vi "welcome.vi"() -> ()   [LabVIEW 2017]
uses:
  GLOBAL/auto.vi
  GLOBAL/all vi close.vi
panel:
  out "first time direct auto":bool
  in  "error in":errorcluster
  in  "EXIT":bool
  in  "PRINTER":bool
  in  "DATA\nHISTORY":bool
  in  "MAIN":bool
  in  "LOGOUT":bool
  in  "USER":bool
  in  "COUNTER":bool
  in  "SETTING":bool
  in  "SHIFT SETTING":bool
  in  "LOGIN":bool
  # "TRACEABILITY"
  # "Powered By- NI Vision, Pune"
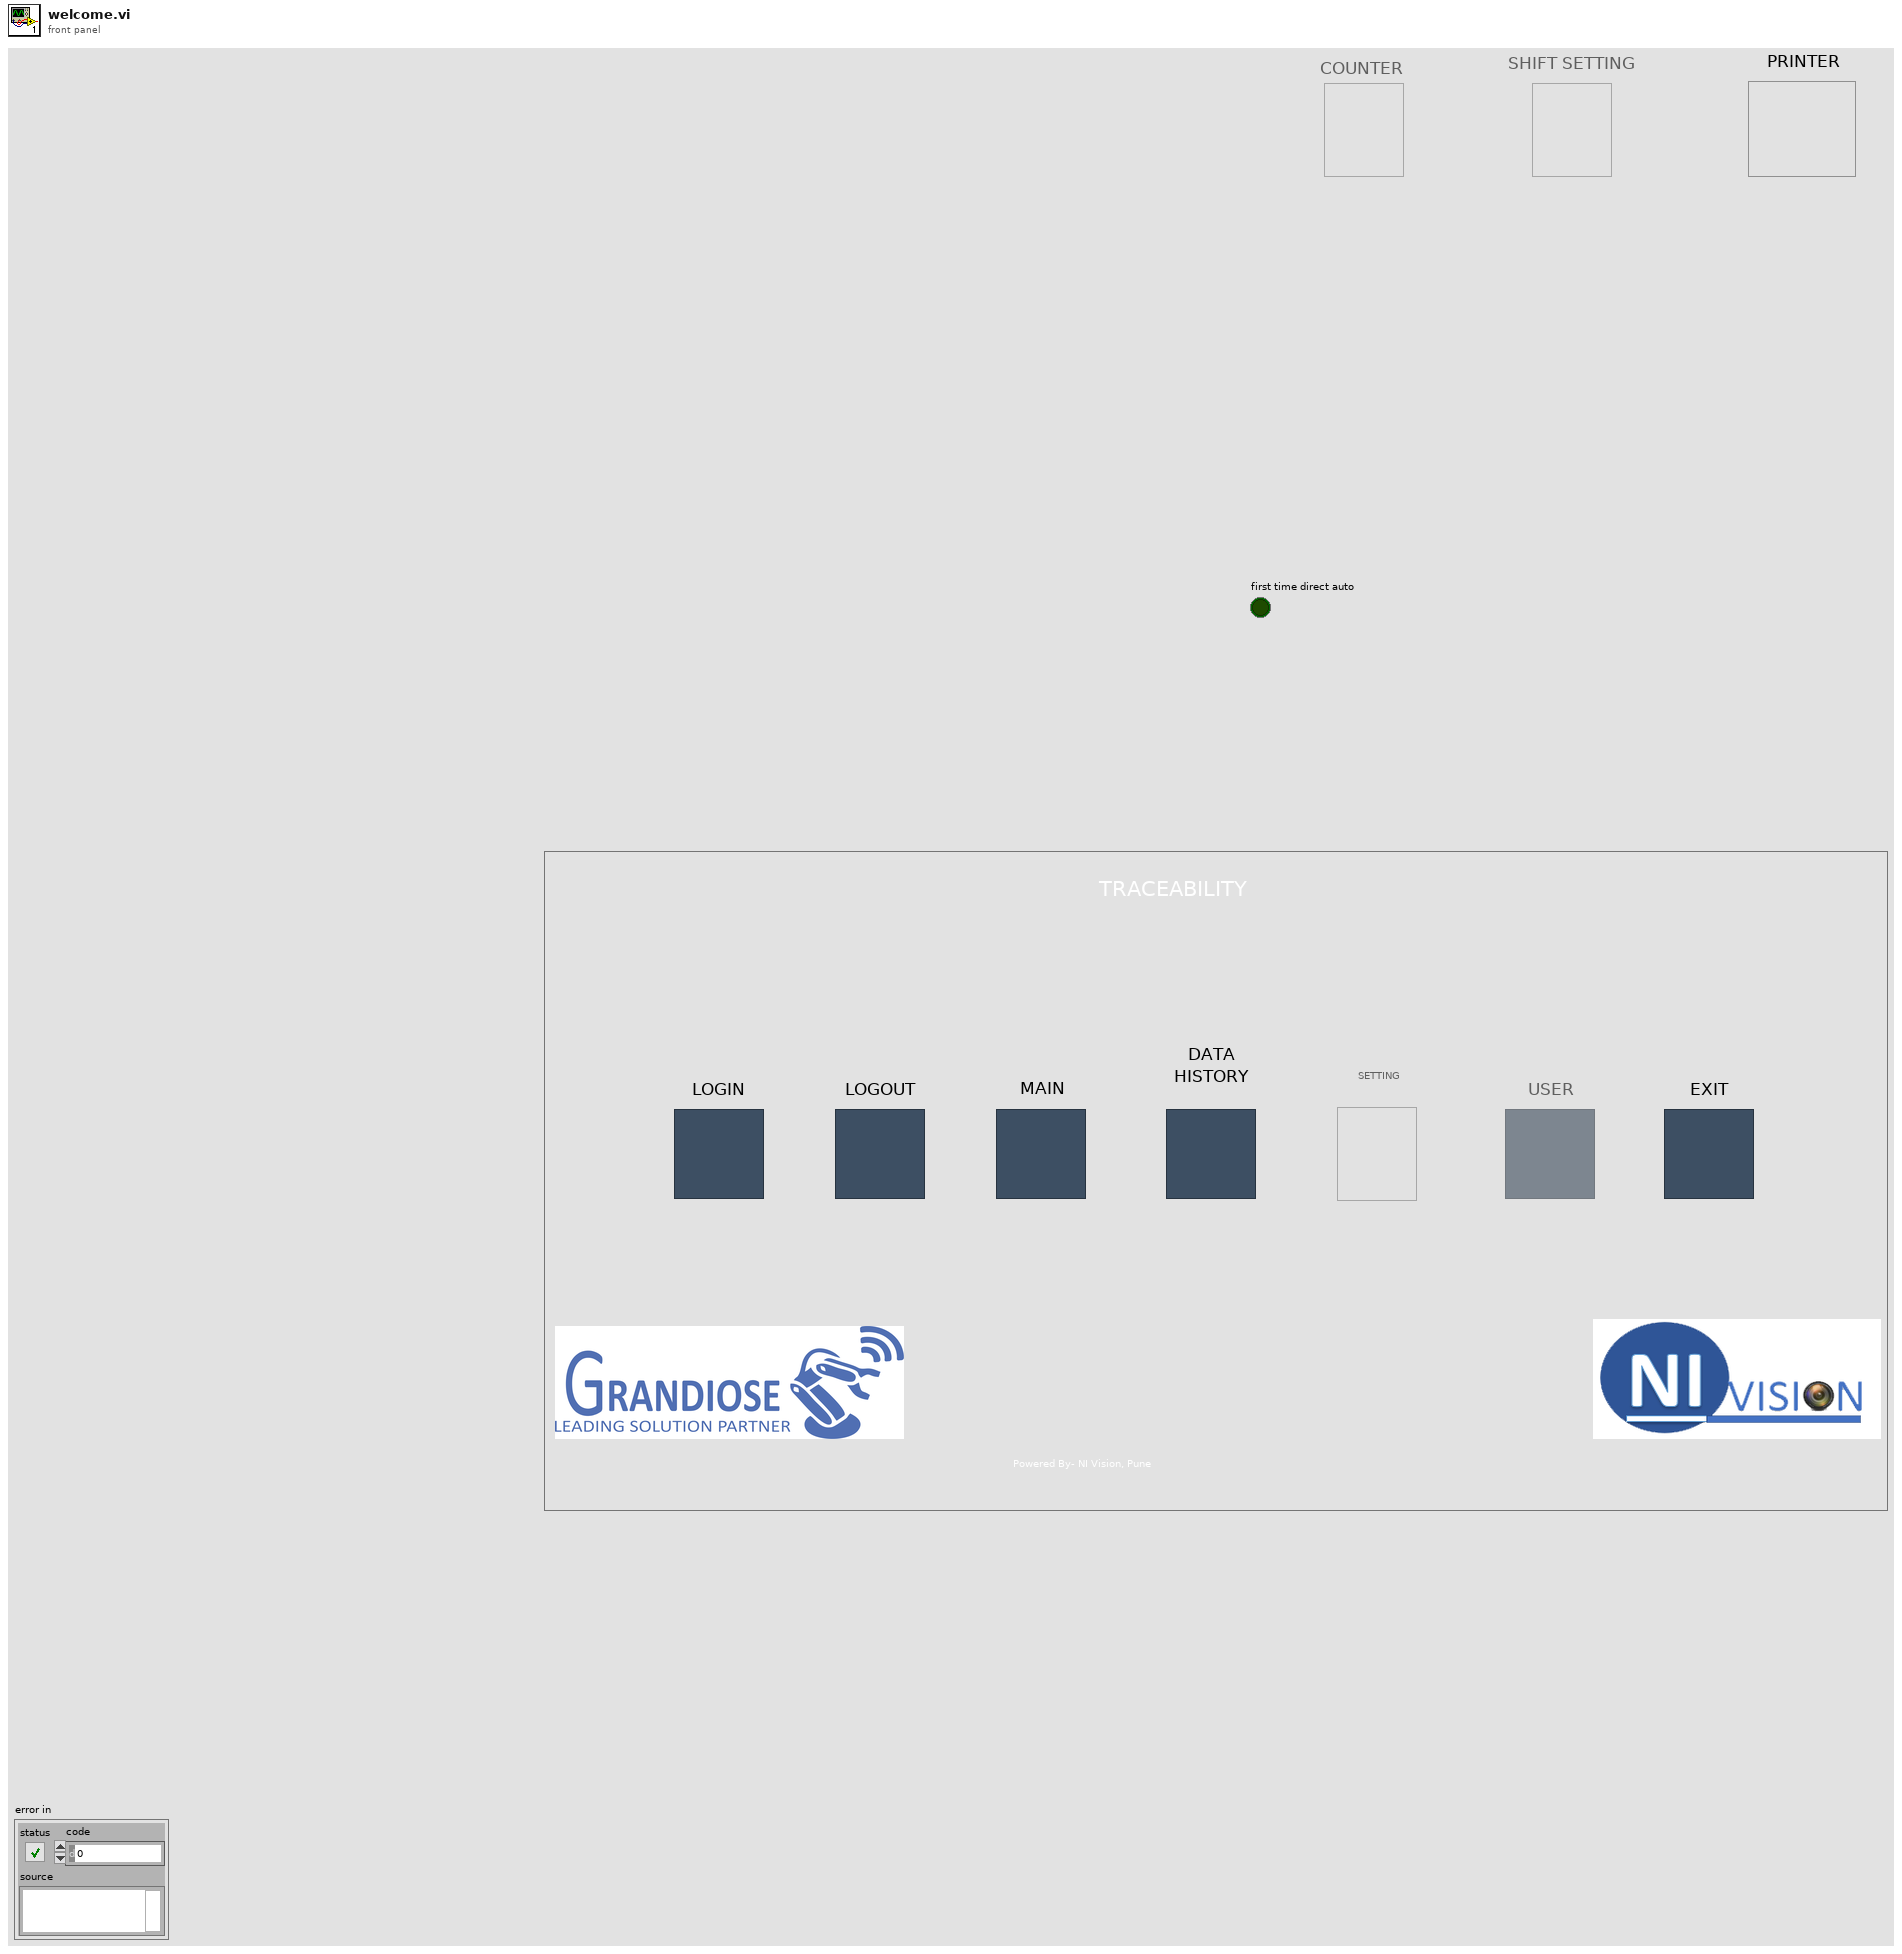
[diagram p1: front panel]
types:
  T1 = enum8{"Enabled", "Disabled", "Disabled and Grayed Out"}
  T2 = enum32{"Invalid", "Standard", "Closed", "Hidden", "Minimized", "Maximized"}
  T3 = enum32{"invalid app kind", "Development System", "Run Time System", "Student Edition", "Embedded LabVIEW", "Evaluation", "Custom"}
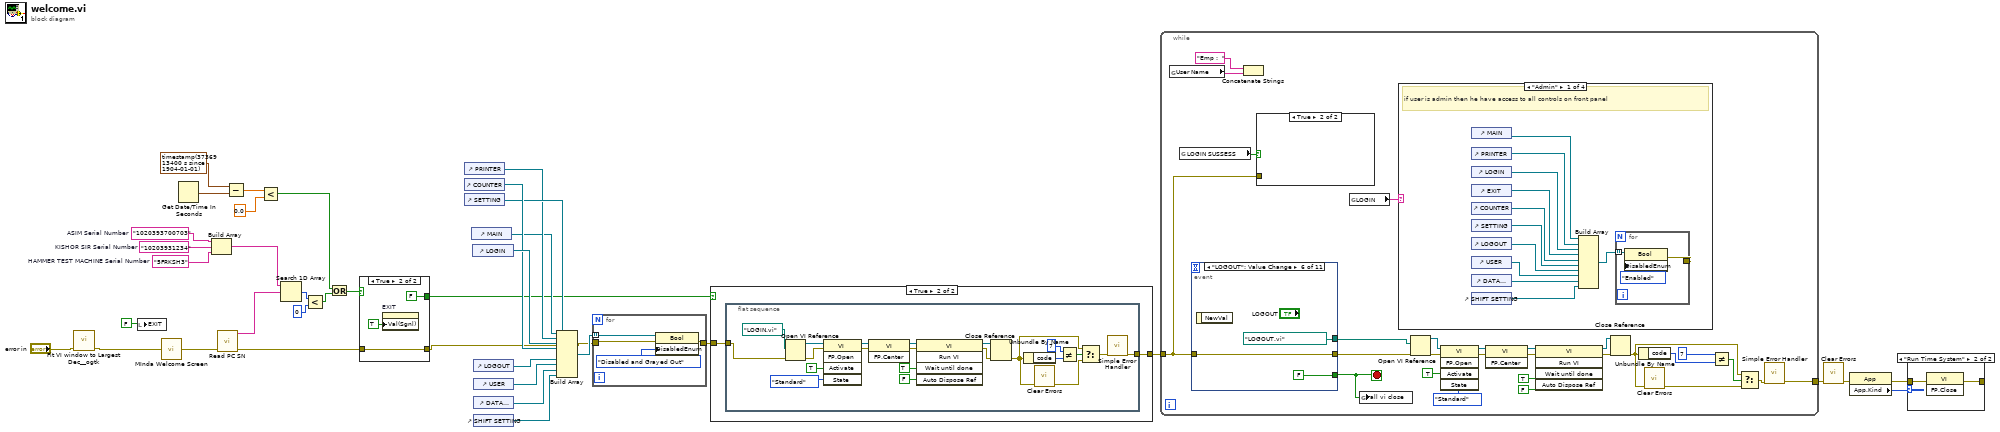
[diagram p0: block diagram]
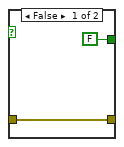
[diagram p3: hidden frame]
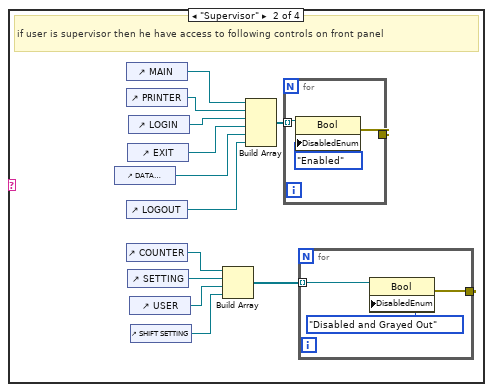
[diagram p6: hidden frame]
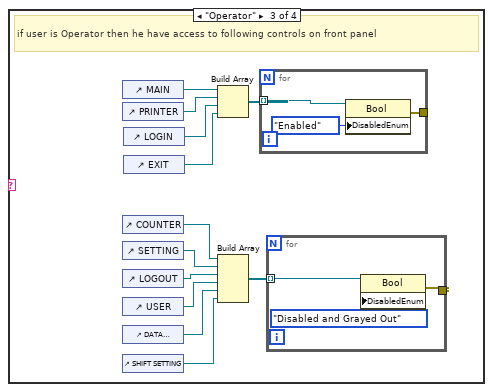
[diagram p7: hidden frame]
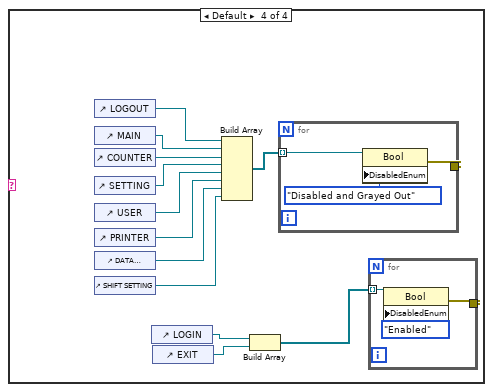
[diagram p8: hidden frame]
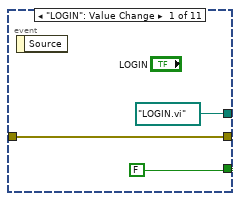
[diagram p9: hidden frame]
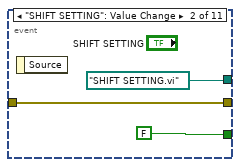
[diagram p10: hidden frame]
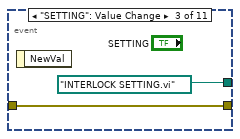
[diagram p11: hidden frame]
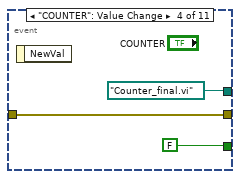
[diagram p12: hidden frame]
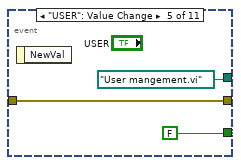
[diagram p13: hidden frame]
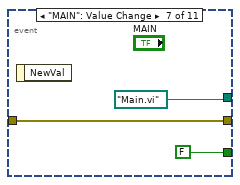
[diagram p14: hidden frame]
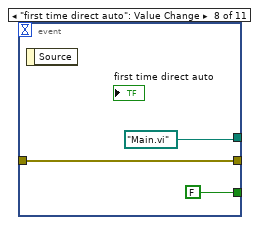
[diagram p15: hidden frame]
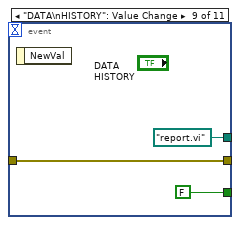
[diagram p16: hidden frame]
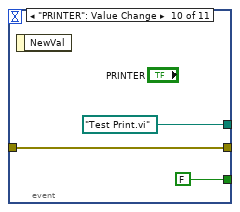
[diagram p17: hidden frame]
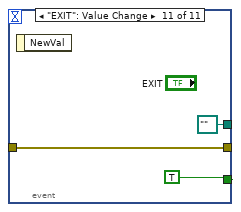
[diagram p18: hidden frame]
diagram:
  w16 = "5FRKSH3"  # HAMMER TEST MACHINE Serial Number
  w17 = "10203931234"  # KISHOR SIR Serial Number
  w18 = "1020393700703"  # ASIM Serial Number
  n1 = call <userlib>:"Fit VI window to Largest Dec__ogtk.vi"("error in (no error)"="error in") -> ("error out"=w10:errorcluster)  [unwired: 5 in, 1 out]
  n2 = local write "EXIT"(FALSE) -> ()
  n3 = call "MInda Welcome Screen.vi"("error in"=w10) -> ("error out"=w20:errorcluster)
  n4 = Get Date/Time In Seconds() -> (seconds since 1Jan1904=w8:timestamp)
  n5 = Build Array(w18, w17, w16) -> (w15:string[])
  n6 = call "Read PC SN.vi"("error in (no error)"=w20) -> ("error out"=w14:errorcluster, "Serial Number"=w19:string)  [unwired: 9 in]
  n7 = Subtract(x=timestamp(3736913400 s since 1904-01-01) ("time stamp"), y=w8) -> (x-y=w7:dbl)
  n8 = Less?(x=w7, y=0.0) -> (x < y?=w1:bool)
  n9 = Search 1D Array(1D array=w15, element=w19) -> (index of element=w5:i32)  [unwired: 1 in]
  n10 = Less?(x=w5, y=0) -> (x < y?=w2:bool)
  n11 = Or(x=w1, y=w2) -> (x .or. y?=w3:bool)
  n12 = case shown="True" w3 {
    tunnel: [w39 w41] -> w13
    tunnel: w14 -> [w39 w41]
    tunnel: [FALSE FALSE] -> w12
    frame False {
    }
    frame True {
      n13 = property on="EXIT" class="Bool (strict)"("Val(Sgnl)"=TRUE) -> ()  [unwired: 2 in, 2 out]
    }
  }
  n14 = control-ref of="PRINTER"() -> (w23:refnum<vi>)
  n15 = control-ref of="COUNTER"() -> (w29:refnum<vi>)
  n16 = control-ref of="SETTING"() -> (w28:refnum<vi>)
  n17 = control-ref of="MAIN"() -> (w22:refnum<vi>)
  n18 = control-ref of="LOGIN"() -> (w30:refnum<vi>)
  n19 = control-ref of="LOGOUT"() -> (w27:refnum<vi>)
  n20 = control-ref of="USER"() -> (w26:refnum<vi>)
  n21 = control-ref of="DATA\nHISTORY"() -> (w25:refnum<vi>)
  n22 = control-ref of="SHIFT SETTING"() -> (w24:refnum<vi>)
  n23 = Build Array(w22, w23, w30, w29, w28, w27, w26, w25, w24) -> (w31:refnum<vi>[])
  n24 = for {
    tunnel: w31 -> [w46] mode=indexing
    tunnel: w13 -> [w44]
    tunnel: [w43] -> w21
    n25 = property class="Bool"(reference=w46, error in=w44, "DisabledEnum"=T1."Disabled and Grayed Out" ("Disabled")) -> (error out=w43:errorcluster)  [unwired: 1 out]
  }
  n26 = case shown="True" w12 {
    tunnel: [w47 w49] -> w36
    tunnel: w21 -> [w47 w48]
    frame False {
    }
    frame True {
      n27 = flat-sequence {
        tunnel: [w51] -> w49
        tunnel: w48 -> [w50]
        frame #0 {
          n28 = Open VI Reference(vi path=path "LOGIN.vi", error in (no error)=w50) -> (vi reference=w58:refnum<vi>, error out=w70:errorcluster)  [unwired: 4 in]
          n29 = invoke class="VI" method="FP.Open"(reference=w58, error in=w70, "Activate"=TRUE ("Activate?"), "State"=T2."Standard") -> (reference out=w69:refnum<vi>, error out=w64:errorcluster)  [unwired: 1 in, 3 out]
          n30 = invoke class="VI" method="FP.Center"(reference=w69, error in=w64) -> (reference out=w65:refnum<vi>, error out=w66:errorcluster)  [unwired: 1 in, 1 out]
          n31 = invoke class="VI" method="Run VI"(reference=w65, error in=w66, "Wait until done"=TRUE ("Wait Until Done"), "Auto Dispose Ref"=FALSE ("Auto Dispose Reference")) -> (reference out=w67:refnum<vi>, error out=w68:errorcluster)  [unwired: 1 in, 3 out]
          n32 = Close Reference(reference=w67, error in (no error)=w68) -> (error out=w59:errorcluster)
          n33 = Unbundle By Name(w59) -> ("code"=w63:i32)
          n34 = call <vilib>:"Clear Errors.vi"("error in (no error)"=w59) -> ("error out"=w61:errorcluster)  [unwired: 5 in, 1 out]
          n35 = Not Equal?(x=7, y=w63) -> (x != y?=w62:bool)
          n36 = Select(t=w59, s=w62, f=w61) -> (s? t:f=w60:errorcluster)
          n37 = call <vilib>:"Simple Error Handler.vi"("error in (no error)"=w60) -> ("error out"=w51:errorcluster)  [unwired: 4 in, 4 out]
        }
      }
    }
  }
  n38 = while {
    tunnel: w36 -> [w73]
    tunnel: [w77] -> w37
    stop <- w75 stop-if-true
    n39 = global read "auto.vi" "User Name"() -> (w72:string)
    n40 = global read "auto.vi" "LOGIN SUSSESS"() -> (w74:bool)
    n41 = event shown="[5] \"LOGOUT\": Value Change" {
      selector: _ -> [_ _ _ _ _ _ _ _ _ _ _]
      dyn-events: _ -> [_ _ _ _ _ _ _ _ _ _ _]
      timeout: _ -> [_ _ _ _ _ _ _ _ _ _ _]
      tunnel: [FALSE FALSE _ FALSE FALSE FALSE FALSE FALSE FALSE FALSE TRUE] -> w75
      tunnel: [path "LOGIN.vi" ("vi path") path "SHIFT SETTING.vi" ("vi path") path "INTERLOCK SETTING.vi" ("vi path") path "Counter_final.vi" ("vi path") path "User mangement.vi" ("vi path") path "LOGOUT.vi" ("vi path") path "Main.vi" ("vi path") path "Main.vi" ("vi path") path "report.vi" ("vi path") path "Test Print.vi" ("vi path") path "" ("vi path")] -> w78
      tunnel: w73 -> [w167 w171 w173 w174 w177 w180 w184 w187 w189 w192 w196]
      tunnel: [w167 w171 w173 w174 w177 w180 w184 w187 w189 w192 w196] -> w79
      event "LOGIN": Value Change {
        n42 = event-data() -> ()  [unwired: 1 in, 1 out]
      }
      event "SHIFT SETTING": Value Change {
        n43 = event-data() -> ()  [unwired: 1 in, 1 out]
      }
      event "SETTING": Value Change {
        n44 = event-data() -> ()  [unwired: 1 in, 1 out]
      }
      event "COUNTER": Value Change {
        n45 = event-data() -> ()  [unwired: 1 in, 1 out]
      }
      event "USER": Value Change {
        n46 = event-data() -> ()  [unwired: 1 in, 1 out]
      }
      event "LOGOUT": Value Change {
        n47 = event-data() -> ()  [unwired: 1 in, 1 out]
      }
      event "MAIN": Value Change {
        n48 = event-data() -> ()  [unwired: 1 in, 1 out]
      }
      event "first time direct auto": Value Change {
        n49 = event-data() -> ()  [unwired: 1 in, 1 out]
      }
      event "DATA\nHISTORY": Value Change {
        n50 = event-data() -> ()  [unwired: 1 in, 1 out]
      }
      event "PRINTER": Value Change {
        n51 = event-data() -> ()  [unwired: 1 in, 1 out]
      }
      event "EXIT": Value Change {
        n52 = event-data() -> ()  [unwired: 1 in, 1 out]
      }
    }
    n53 = Concatenate Strings("Emp :  " ("string"), w72) -> ()  [unwired: 1 out]
    n54 = case shown="True" w74 {
      tunnel: w73 -> [_ _]
      frame False {
      }
      frame True {
      }
    }
    n55 = global read "auto.vi" "LOGIN"() -> (w76:string)
    n56 = global write "all vi close.vi" "all vi close"(w75) -> ()
    n57 = case shown="\"Admin\"" w76 {
      frame "Admin" {
        # "if user is admin then he have access to all controls on front panel"
        n58 = control-ref of="MAIN"() -> (w98:refnum<vi>)
        n59 = control-ref of="PRINTER"() -> (w99:refnum<vi>)
        n60 = control-ref of="LOGIN"() -> (w107:refnum<vi>)
        n61 = control-ref of="EXIT"() -> (w106:refnum<vi>)
        n62 = control-ref of="COUNTER"() -> (w105:refnum<vi>)
        n63 = control-ref of="SETTING"() -> (w104:refnum<vi>)
        n64 = control-ref of="LOGOUT"() -> (w103:refnum<vi>)
        n65 = control-ref of="USER"() -> (w102:refnum<vi>)
        n66 = control-ref of="DATA\nHISTORY"() -> (w101:refnum<vi>)
        n67 = control-ref of="SHIFT SETTING"() -> (w100:refnum<vi>)
        n68 = Build Array(w98, w99, w107, w106, w105, w104, w103, w102, w101, w100) -> (w108:refnum<vi>[])
        n69 = for {
          tunnel: w108 -> [w109] mode=indexing
          tunnel: [w110] -> _
          n70 = property class="Bool"(reference=w109, "DisabledEnum"=T1."Enabled" ("Disabled")) -> (error out=w110:errorcluster)  [unwired: 1 in, 1 out]
        }
      }
      frame "Supervisor" {
        # "if user is supervisor then he have access to following controls on front panel"
        n71 = control-ref of="DATA\nHISTORY"() -> (w119:refnum<vi>)
        n72 = control-ref of="MAIN"() -> (w112:refnum<vi>)
        n73 = control-ref of="PRINTER"() -> (w113:refnum<vi>)
        n74 = control-ref of="LOGOUT"() -> (w118:refnum<vi>)
        n75 = control-ref of="COUNTER"() -> (w117:refnum<vi>)
        n76 = control-ref of="EXIT"() -> (w120:refnum<vi>)
        n77 = control-ref of="SETTING"() -> (w116:refnum<vi>)
        n78 = control-ref of="LOGIN"() -> (w121:refnum<vi>)
        n79 = control-ref of="USER"() -> (w115:refnum<vi>)
        n80 = control-ref of="SHIFT SETTING"() -> (w114:refnum<vi>)
        n81 = Build Array(w117, w116, w115, w114) -> (w122:refnum<vi>[])
        n82 = Build Array(w112, w113, w121, w120, w119, w118) -> (w123:refnum<vi>[])
        n83 = for {
          tunnel: w123 -> [w127] mode=indexing
          tunnel: [w128] -> _
          n84 = property class="Bool"(reference=w127, "DisabledEnum"=T1."Enabled" ("Disabled")) -> (error out=w128:errorcluster)  [unwired: 1 in, 1 out]
        }
        n85 = for {
          tunnel: [w125] -> _
          tunnel: w122 -> [w124] mode=indexing
          n86 = property class="Bool"(reference=w124, "DisabledEnum"=T1."Disabled and Grayed Out" ("Disabled")) -> (error out=w125:errorcluster)  [unwired: 1 in, 1 out]
        }
      }
      frame "Operator" {
        # "if user is Operator then he have access to following controls on front panel"
        n87 = control-ref of="MAIN"() -> (w130:refnum<vi>)
        n88 = control-ref of="PRINTER"() -> (w139:refnum<vi>)
        n89 = control-ref of="COUNTER"() -> (w133:refnum<vi>)
        n90 = control-ref of="SETTING"() -> (w138:refnum<vi>)
        n91 = control-ref of="LOGOUT"() -> (w137:refnum<vi>)
        n92 = control-ref of="USER"() -> (w136:refnum<vi>)
        n93 = control-ref of="DATA\nHISTORY"() -> (w135:refnum<vi>)
        n94 = control-ref of="SHIFT SETTING"() -> (w134:refnum<vi>)
        n95 = control-ref of="LOGIN"() -> (w132:refnum<vi>)
        n96 = control-ref of="EXIT"() -> (w131:refnum<vi>)
        n97 = Build Array(w130, w139, w132, w131) -> (w141:refnum<vi>[])
        n98 = Build Array(w133, w138, w137, w136, w135, w134) -> (w140:refnum<vi>[])
        n99 = for {
          tunnel: w141 -> [w147] mode=indexing
          tunnel: [w145] -> _
          n100 = property class="Bool"(reference=w147, "DisabledEnum"=T1."Enabled" ("Disabled")) -> (error out=w145:errorcluster)  [unwired: 1 in, 1 out]
        }
        n101 = for {
          tunnel: w140 -> [w144] mode=indexing
          tunnel: [w142] -> _
          n102 = property class="Bool"(reference=w144, "DisabledEnum"=T1."Disabled and Grayed Out" ("Disabled")) -> (error out=w142:errorcluster)  [unwired: 1 in, 1 out]
        }
      }
      frame Default {
        n103 = control-ref of="LOGOUT"() -> (w152:refnum<vi>)
        n104 = control-ref of="MAIN"() -> (w151:refnum<vi>)
        n105 = control-ref of="COUNTER"() -> (w153:refnum<vi>)
        n106 = control-ref of="SETTING"() -> (w154:refnum<vi>)
        n107 = control-ref of="USER"() -> (w155:refnum<vi>)
        n108 = control-ref of="PRINTER"() -> (w156:refnum<vi>)
        n109 = control-ref of="DATA\nHISTORY"() -> (w157:refnum<vi>)
        n110 = control-ref of="SHIFT SETTING"() -> (w158:refnum<vi>)
        n111 = control-ref of="LOGIN"() -> (w148:refnum<vi>)
        n112 = control-ref of="EXIT"() -> (w150:refnum<vi>)
        n113 = Build Array(w152, w151, w153, w154, w155, w156, w157, w158) -> (w159:refnum<vi>[])
        n114 = Build Array(w148, w150) -> (w149:refnum<vi>[])
        n115 = for {
          tunnel: w159 -> [w163] mode=indexing
          tunnel: [w164] -> _
          n116 = property class="Bool"(reference=w163, "DisabledEnum"=T1."Disabled and Grayed Out" ("Disabled")) -> (error out=w164:errorcluster)  [unwired: 1 in, 1 out]
        }
        n117 = for {
          tunnel: w149 -> [w160] mode=indexing
          tunnel: [w161] -> _
          n118 = property class="Bool"(reference=w160, "DisabledEnum"=T1."Enabled" ("Disabled")) -> (error out=w161:errorcluster)  [unwired: 1 in, 1 out]
        }
      }
    }
    n119 = Open VI Reference(vi path=w78, error in (no error)=w79) -> (vi reference=w97:refnum<vi>, error out=w86:errorcluster)  [unwired: 4 in]
    n120 = invoke class="VI" method="FP.Open"(reference=w97, error in=w86, "Activate"=TRUE ("Activate?"), "State"=T2."Standard") -> (reference out=w87:refnum<vi>, error out=w92:errorcluster)  [unwired: 1 in, 3 out]
    n121 = invoke class="VI" method="FP.Center"(reference=w87, error in=w92) -> (reference out=w91:refnum<vi>, error out=w90:errorcluster)  [unwired: 1 in, 1 out]
    n122 = invoke class="VI" method="Run VI"(reference=w91, error in=w90, "Wait until done"=TRUE ("Wait Until Done"), "Auto Dispose Ref"=FALSE ("Auto Dispose Reference")) -> (reference out=w89:refnum<vi>, error out=w88:errorcluster)  [unwired: 1 in, 3 out]
    n123 = Close Reference(reference=w89, error in (no error)=w88) -> (error out=w85:errorcluster)
    n124 = Unbundle By Name(w85) -> ("code"=w93:i32)
    n125 = call <vilib>:"Clear Errors.vi"("error in (no error)"=w85) -> ("error out"=w95:errorcluster)  [unwired: 5 in, 1 out]
    n126 = Not Equal?(x=7, y=w93) -> (x != y?=w94:bool)
    n127 = Select(t=w85, s=w94, f=w95) -> (s? t:f=w96:errorcluster)
    n128 = call <vilib>:"Simple Error Handler.vi"("error in (no error)"=w96) -> ("error out"=w77:errorcluster)  [unwired: 4 in, 4 out]
  }
  n129 = call <vilib>:"Clear Errors.vi"("error in (no error)"=w37) -> ("error out"=w33:errorcluster)  [unwired: 5 in, 1 out]
  n130 = property class="App"(error in=w33) -> (error out=w34:errorcluster, "App.Kind"=w35:T3)  [unwired: 1 in, 1 out]
  n131 = case shown="\"Run Time System\"" w35 {
    tunnel: w34 -> [w198 w200]
    tunnel: [w198 w199] -> _
    frame Default {
    }
    frame "Run Time System" {
      n132 = invoke class="VI" method="FP.Close"(error in=w200) -> (error out=w199:errorcluster)  [unwired: 2 in, 2 out]
    }
  }
